vi "ClearOTP.vi"(8 "error in (no error)":errorcluster caption="错误输入（无错误）", 11 "SENSOR":T1) -> (0 "error out":errorcluster caption="错误输出")   [LabVIEW 2020]
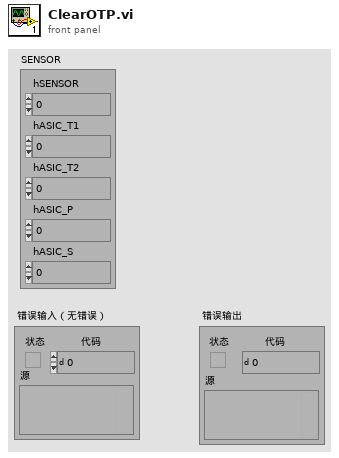
[diagram p1: front panel]
types:
  T1 = cluster{"hSENSOR":i32, "hASIC_T1":i32, "hASIC_T2":i32, "hASIC_P":i32, "hASIC_S":i32}
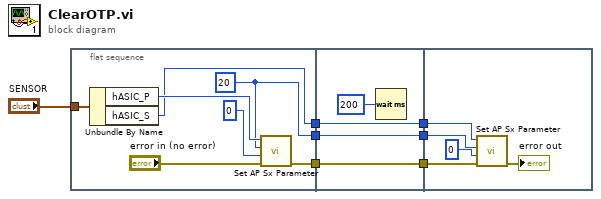
[diagram p0: block diagram]
diagram:
  n1 = flat-sequence {
    tunnel: "SENSOR" -> [w14]
    tunnel: [w12] -> w7
    tunnel: [w10] -> w6
    tunnel: [w9] -> w5
    tunnel: w7 -> [w18]
    tunnel: [w18] -> w4
    tunnel: w6 -> [w17]
    tunnel: [w17] -> w3
    tunnel: w5 -> [w16]
    tunnel: [w16] -> w2
    tunnel: w4 -> [w23]
    tunnel: w3 -> [w22]
    tunnel: w2 -> [w21]
    frame #0 {
      w10 = 20 ("asicBitsName")
      n2 = Unbundle By Name(w14) -> ("hASIC_P"=w13:i32, "hASIC_S"=w9:i32)
      n3 = call "Set AP Sx Parameter.vi"("error in (no error)"="error in (no error)", "para2"=0, "asicBitsName"=w10, "asicHandle"=w13) -> ("error out"=w12:errorcluster)  [unwired: 6 in, 1 out]
    }
    frame #1 {
      n4 = Wait (ms)(milliseconds to wait=u32 200 ("等待时间（毫秒）")) -> ()  [unwired: 1 out]
    }
    frame #2 {
      n5 = call "Set AP Sx Parameter.vi"("error in (no error)"=w23, "para2"=0, "asicBitsName"=w22, "asicHandle"=w21) -> ("error out"=→"error out":errorcluster)  [unwired: 6 in, 1 out]
    }
  }
